vi "solar_voy Packet Unpack.vi"(6 "Suppress Errors? (T)":bool=TRUE, 8 "error in (no error)":errorcluster, 10 "TCP Message Read":string, 11 "PACKET in":T1 {"last_time" format="%<%H:%M:%S%3u %m/%d/%y>T"}) -> (0 "error out":errorcluster, 1 "Item Values (TCP)":string[](array[string]), 2 "Item Values":variant[](array[variant]), 3 "PACKET out":T1 {"last_time" format="%<%H:%M:%S%3u %m/%d/%y>T"})   [LabVIEW 2018]
doc: "This unpacks a TCP message into the packet definition. All values are converted into LabVIEW native data types."
uses:
  solar_voy_def_ctl ITEM TYPE.ctl
  type/solar_type Item Type.ctl
  solar_voy_def_ctl ITEM.ctl
  solar_voy_def_ctl PACKET.ctl
  solar_voy_def_ctl PACKET_ID.ctl
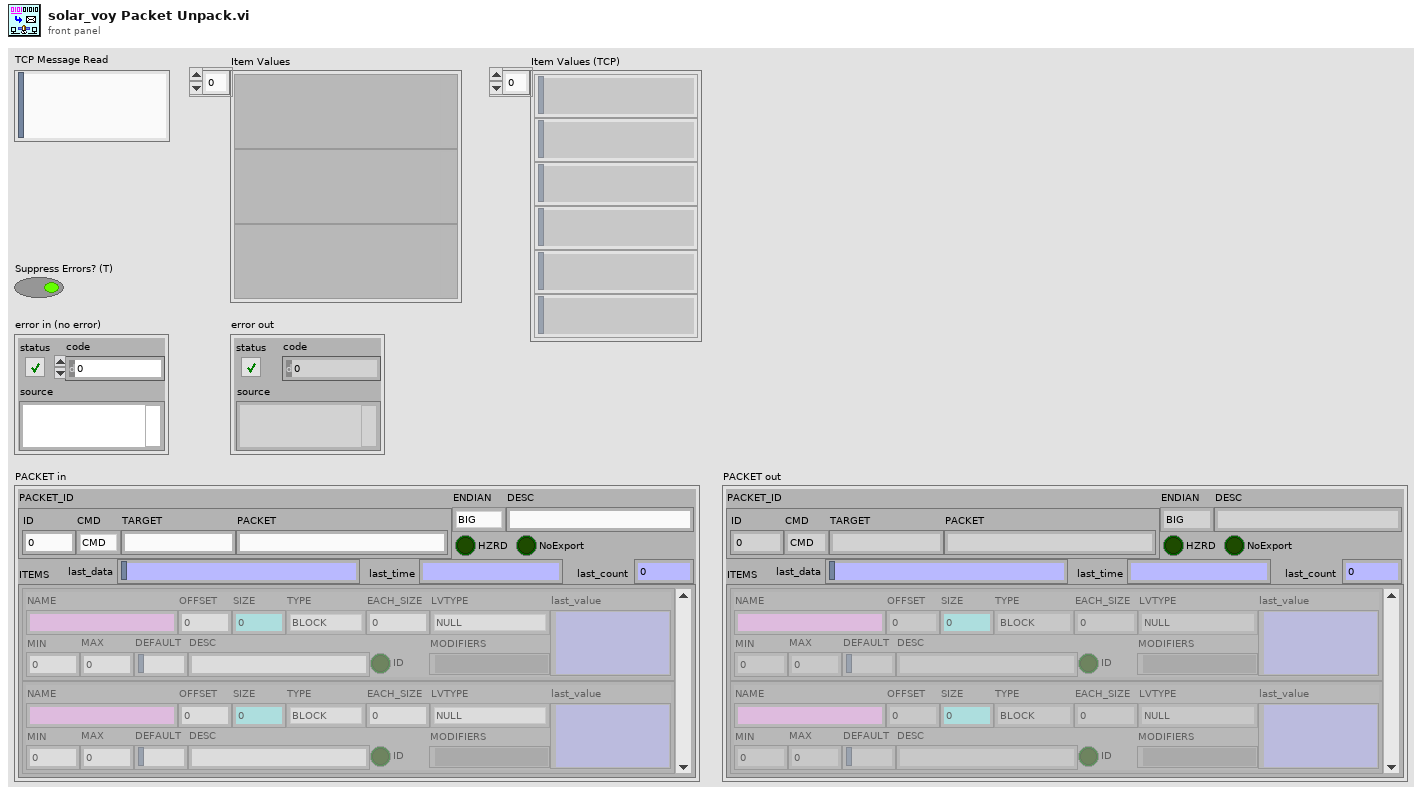
[diagram p1: front panel]
types:
  T1 = typedef "solar_voy_def_ctl PACKET.ctl" = cluster{"PACKET_ID":T2, "ENDIAN":enum8{"BIG", "LITTLE"}, "DESC":string, "HZRD":bool, "ITEMS":T3[], "NoExport":bool, "last_time":timestamp, "last_count":u32, "last_data":string}
  T2 = typedef "solar_voy_def_ctl PACKET_ID.ctl" = cluster{"ID":u16, "CMD":enum8{"CMD", "TLM"}, "TARGET":string, "PACKET":string}
  T3 = typedef "solar_voy_def_ctl ITEM.ctl" = cluster{"NAME":string, "OFFSET":i32, "SIZE":i32, "TYPE":T4, "EACH_SIZE":i32, "LVTYPE":T5, "MIN":dbl, "MAX":dbl, "DEFAULT":string, "DESC":string, "ID":bool, "MODIFIERS":variant, "last_value":variant}
  T4 = typedef "solar_voy_def_ctl ITEM TYPE.ctl" = enum8{"BLOCK", "INT", "UINT", "FLOAT", "STRING"}
  T5 = typedef "solar_type Item Type.ctl" = enum16{"NULL", "UNKNOWN", "CLUSTER", "I8", "I16", "I32", "I64", "U8", "U16", "U32", "U64", "U8_ENUM", "U16_ENUM", "U32_ENUM", "SGL", "DBL", "BOOLEAN", "STRING", "PATH", "VISA", "TAG", "TIME", "I8_1D", "I16_1D", "I32_1D", "I64_1D", "U8_1D", "U16_1D", "U32_1D", "U64_1D", "U8_ENUM_1D", "U16_ENUM_1D", "U32_ENUM_1D", "SGL_1D", "DBL_1D", "BOOLEAN_1D", "STRING_1D", "PATH_1D", "VISA_1D", "TAG_1D", "TIME_1D", "I8_2D", "I16_2D", "I32_2D", "I64_2D", "U8_2D", "U16_2D", "U32_2D", "U64_2D", "U8_ENUM_2D", "U16_ENUM_2D", "U32_ENUM_2D", "SGL_2D", "DBL_2D", "BOOLEAN_2D", "STRING_2D", "PATH_2D", "VISA_2D", "TAG_2D", "TIME_2D"}
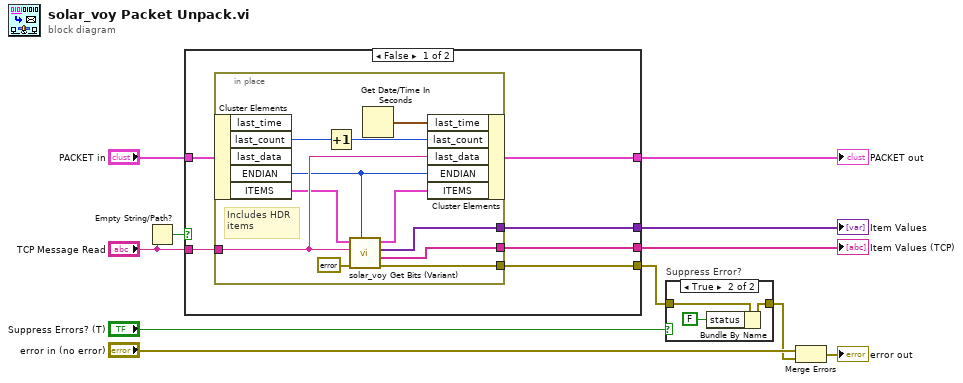
[diagram p0: block diagram]
diagram:
  n1 = Empty String/Path?(string/path="TCP Message Read") -> (empty?=w3:bool)
  n2 = case shown="False" w3 {
    tunnel: "PACKET in" -> [w15 w29]
    tunnel: "TCP Message Read" -> [w16 _]
    tunnel: [w17 _] -> w6
    tunnel: [w14 w29] -> w5
    tunnel: [w13 _] -> w2
    tunnel: [w12 _] -> w1
    frame False {
      n3 = in-place {
        in-place-border: [w27] -> w17
        in-place-border: [w26] -> w13
        in-place-border: w16 -> [w22]
        in-place-border: [w18] -> w12
        # "Includes HDR\nitems"
        n4 = in-place-cluster #1(w15) -> ("last_count"=w24:u32, "ENDIAN"=w19:enum8{"BIG", "LITTLE"}, "ITEMS"=w20:T3[])  [unwired: 2 out]
        n5 = Increment(x=w24) -> (x+1=w23:u32)
        n6 = call "solar_voy Get Bits (Variant).vi"("Endian (BIG)"=w19, "error in (no error)"=errorcluster {"status"=FALSE, "code"=0, "source"=""}, "COSMOS Data"=w22, "ITEMS in"=w20) -> ("error out"=w27:errorcluster, "Item Values (LV Flattened Value)"=w18:string[], "Item Values"=w26:variant[], "ITEMS out"=w21:T3[])  [unwired: 4 in]
        n7 = Get Date/Time In Seconds() -> (seconds since 1Jan1904=w25:timestamp)
        n8 = in-place-cluster #1("last_time"=w25, "last_count"=w23, "last_data"=w22, "ENDIAN"=w19, "ITEMS"=w21) -> (w14:T1)
      }
    }
    frame True {
      # "Invalid data"
    }
  }
  "PACKET out" <- w5
  "Item Values" <- w2
  "Item Values (TCP)" <- w1
  n9 = case "Suppress Error?" shown="True" "Suppress Errors? (T)" {
    tunnel: w6 -> [w30 w33]
    tunnel: [w30 w32] -> w9
    frame False {
    }
    frame True {
      n10 = Bundle By Name(cluster=w33, "status"=FALSE) -> (w32:errorcluster)
    }
  }
  n11 = Merge Errors("error in (no error)", w9) -> (→"error out":errorcluster)
